vi "2d_array_average.vi"(4 "2D array":dbl[][](array[numeric])) -> (1 "array average":dbl[](array[numeric]))   [LabVIEW 2011]
doc: "computes the average over an 2d array"
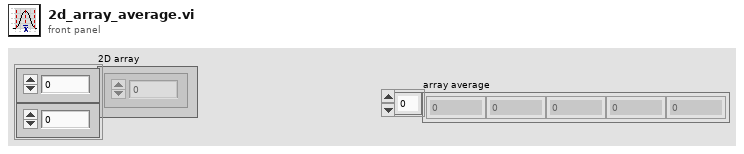
[diagram p1: front panel]
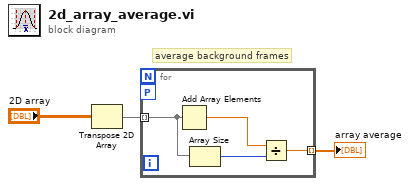
[diagram p0: block diagram]
diagram:
  # "average background frames"
  n1 = Transpose 2D Array(2D array="2D array") -> (transposed array=w2:dbl[][])
  n2 = for {
    tunnel: w2 -> [w5] mode=indexing
    tunnel: [w6] -> w3 mode=indexing
    workers-P: _ -> [_]
    n3 = Add Array Elements(numeric array=w5) -> (sum=w7:dbl)
    n4 = Array Size(array=w5) -> (size(s)=w4:i32)
    n5 = Divide(x=w7, y=w4) -> (x/y=w6:dbl)
  }
  "array average" <- w3
